vi "get_timeout.vi"(0 "HGF_Event.lvclass in":refnum<class "HGF_Event.lvclass">, 5 "error in (no error)":errorcluster) -> (14 "HGF_Event.lvclass out":refnum<class "HGF_Event.lvclass">, 17 "timeout":i32, 19 "error out":errorcluster)   [LabVIEW 2014, in "HGF_BaseClasses.lvlib" / "HGF_Event.lvclass"]
doc: "Get timeout value."
uses:
  HGF_Event.lvclass
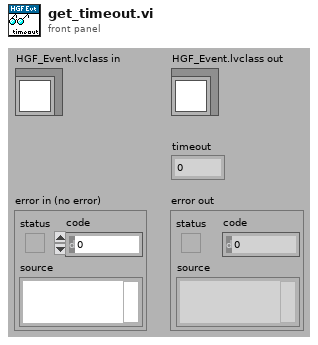
[diagram p1: front panel]
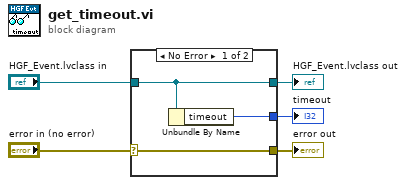
[diagram p0: block diagram]
diagram:
  n1 = case shown="No Error" "error in (no error)" {
    selector: "error in (no error)" -> [w8 w9]
    tunnel: [w8 w9] -> w4
    tunnel: [w7 w10] -> w2
    tunnel: "HGF_Event.lvclass in" -> [w7 w10]
    tunnel: [w6 _] -> w1
    frame No Error {
      n2 = Unbundle By Name(w7) -> ("timeout"=w6:i32)
    }
    frame Error {
    }
  }
  "error out" <- w4
  "HGF_Event.lvclass out" <- w2
  "timeout" <- w1
